vi "Actor Stopped.vi"(8 "error in (no error)":errorcluster, 10 "Actor ID":string, 11 "Actor Monitor in":refnum<class "Actor Monitor.lvclass">) -> (0 "error out":errorcluster, 3 "Actor Monitor out":refnum<class "Actor Monitor.lvclass">)   [LabVIEW 2018, in "Monitored Actor.lvlib" / "Actor Monitor.lvclass"]
doc: "Removed the actor from all data structures.\n\nLookup the Queue value from queue lookup by core name. Delete this value, then use the value to lookup the entry in the nested Actor Lookup Table and delete it.\n\nIf all monitored actors are closed, send a stop message to the UI\n\nCopyright: MGI\nAuthored by: Derek Trepanier"
uses:
  Actor Monitor.lvclass
  C:/Program Files (x86)/National Instruments/LabVIEW 2018/vi.lib/ActorFramework/Actor/Actor.lvclass
  Actor Monitor.lvclass/Actor Monitor.ctl
  <vilib>/ActorFramework/Actor/Actor.lvclass/Actor.ctl
  <vilib>/ActorFramework/Message Enqueuer/Message Enqueuer.lvclass/Message Enqueuer.ctl
  <vilib>/ActorFramework/Message Enqueuer/Init from Existing Queue.vi
  <vilib>/ActorFramework/Message Enqueuer/Enqueue.vi
  <vilib>/ActorFramework/Stop Msg/Stop Msg.lvclass
  C:/Program Files (x86)/National Instruments/LabVIEW 2018/vi.lib/ActorFramework/Message/Message.lvclass
  <vilib>/ActorFramework/Message Priority Queue/Priority Enqueue.vi
  <vilib>/ActorFramework/Message Enqueuer/Message Enqueuer.lvclass
  <vilib>/ActorFramework/Actor/Actor.lvclass
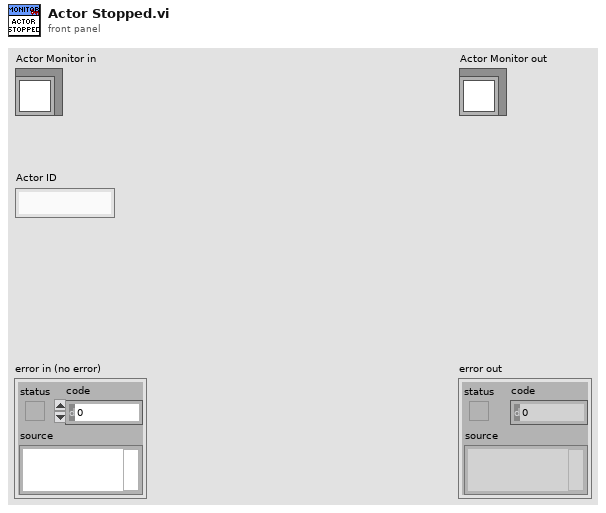
[diagram p1: front panel]
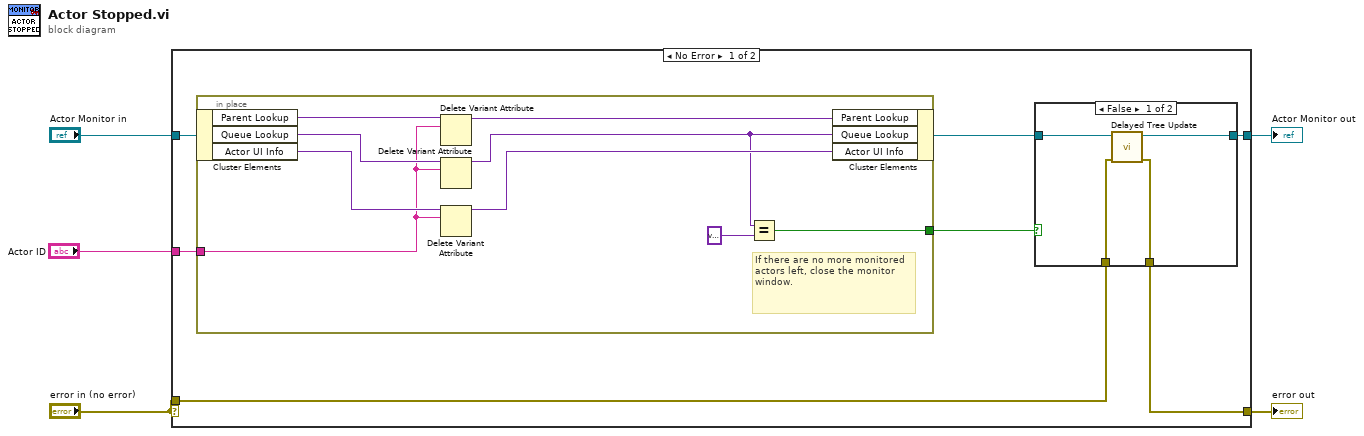
[diagram p0: block diagram]
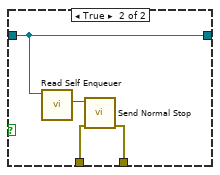
[diagram p2: hidden frame]
diagram:
  n1 = case shown="No Error" "error in (no error)" {
    selector: "error in (no error)" -> [_ w31]
    tunnel: [w6 w31] -> w5
    tunnel: [w9 w30] -> w3
    tunnel: "Actor Monitor in" -> [w12 w30]
    tunnel: "Actor ID" -> [w11 _]
    tunnel: "error in (no error)" -> [w7 _]
    frame No Error {
      n2 = in-place {
        in-place-border: w11 -> [w24]
        in-place-border: [w28] -> w10
        # "If there are no more monitored actors left, close the monitor window."
        n3 = in-place-cluster #1(w12) -> ("Parent Lookup"=w27:variant, "Queue Lookup"=w26:variant, "Actor UI Info"=w25:variant)
        n4 = Delete Variant Attribute(6:w24, 7:w27) -> (3:w23:variant)  [unwired: 1 in, 2 out]
        n5 = Delete Variant Attribute(6:w24, 7:w26) -> (3:w21:variant)  [unwired: 1 in, 2 out]
        n6 = Delete Variant Attribute(6:w24, 7:w25) -> (3:w22:variant)  [unwired: 1 in, 2 out]
        n7 = Equal?(x=w21, y=variant) -> (x = y?=w28:bool)
        n8 = in-place-cluster #1("Parent Lookup"=w23, "Queue Lookup"=w21, "Actor UI Info"=w22) -> (w8:refnum<class "Actor Monitor.lvclass">)
      }
      n9 = case shown="False" w10 {
        tunnel: [w15 w20] -> w9
        tunnel: w8 -> [w16 w20]
        tunnel: w7 -> [w14 w17]
        tunnel: [w13 w18] -> w6
        frame False {
          n10 = call "Delayed Tree Update.vi"("error in (no error)"=w14, "Actor Monitor in"=w16) -> ("error out"=w13:errorcluster, "Actor Monitor out"=w15:refnum<class "Actor Monitor.lvclass">)  [unwired: 8 in]
        }
        frame True {
          n11 = call <vilib>:"Read Self Enqueuer.vi"("Actor"=w20) -> ("Self Enqueuer"=w19:refnum<class "Message Enqueuer.lvclass">)  [unwired: 10 in]
          n12 = call <vilib>:"Send Normal Stop.vi"("error in (no error)"=w17, "Message Enqueuer"=w19) -> ("error out"=w18:errorcluster)  [unwired: 9 in]
        }
      }
    }
    frame Error {
    }
  }
  "error out" <- w5
  "Actor Monitor out" <- w3
